vi "Power, Conserve Sign.vi"(2 "Input":dbl, 3 "Power":dbl=1.0) -> (0 "Output":dbl)   [LabVIEW 2012]
doc: "Raises the <b>input</b> to the specified <b>power</b>, keeping the sign the same as the original. This is useful for tightening joystick control or for modifying waveforms."
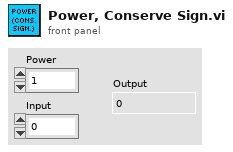
[diagram p1: front panel]
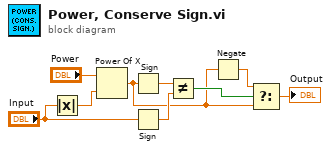
[diagram p0: block diagram]
diagram:
  n1 = Absolute Value(x="Input") -> (abs(x)=w8:dbl)
  n2 = Power Of X(1:w8, 2:"Power") -> (0:w3:dbl)
  n3 = Sign(1:w3) -> (0:w4:dbl)
  n4 = Sign(1:"Input") -> (0:w5:dbl)
  n5 = Not Equal?(x=w4, y=w5) -> (x != y?=w6:bool)
  n6 = Negate(x=w3) -> (-x=w2:dbl)
  n7 = Select(t=w2, s=w6, f=w3) -> (s? t:f=→"Output":dbl)
